vi "Registry WinErr-LVErr.vi"(4 "Windows error":i32) -> (1 "LabVIEW error":i32)   [LabVIEW 2020]
doc: "Maps Windows Registry errors from Windows into LabVIEW errors."
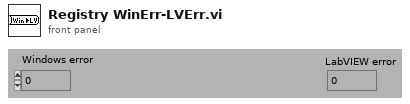
[diagram p1: front panel]
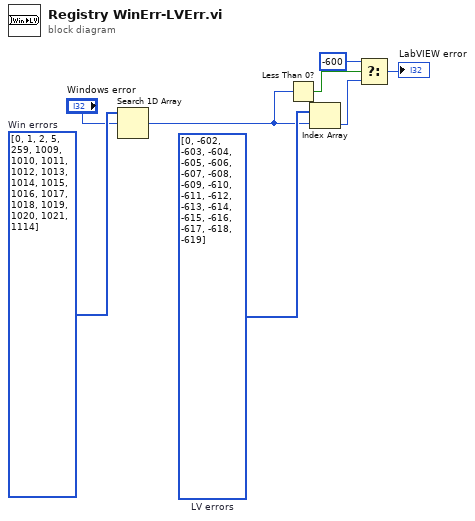
[diagram p0: block diagram]
diagram:
  w7 = i32[] [0, -602, -603, -604, -605, -606, -607, -608, -609, -610, -611, -612, -613, -614, -615, -616, -617, -618, -619]  # LV errors
  w8 = i32[] [0, 1, 2, 5, 259, 1009, 1010, 1011, 1012, 1013, 1014, 1015, 1016, 1017, 1018, 1019, 1020, 1021, 1114]  # Win errors
  n1 = Search 1D Array(1D array=w8, element="Windows error") -> (index of element=w5:i32)  [unwired: 1 out]
  n2 = Less Than 0?(x=w5) -> (x < 0?=w4:bool)
  n3 = Index Array(array=w7, index=w5) -> (element=w2:i32)
  n4 = Select(t=-600, s=w4, f=w2) -> (s? t:f=→"LabVIEW error":i32)
